vi "Logic for Default Case.vi"(11 "error in (no error)":errorcluster) -> (15 "error out":errorcluster)   [LabVIEW 2021, in "Migrator.lvlib"]
uses:
  Migrator.lvlib
  <vilib>/Utility/traverseref.llb/TRef TravTarget.ctl
  <vilib>/Utility/traverseref.llb/VI Scripting - Traverse.lvlib
  Path Functions/Path Functions.lvlib
  Migrator Reusables/Migrator Reusables.lvlib
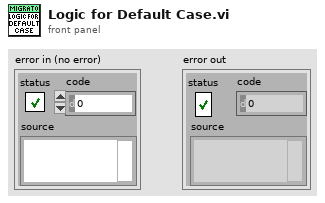
[diagram p1: front panel]
types:
  T1 = typedef "TRef TravTarget.ctl" = enum16{"FP", "BD", "Other"}
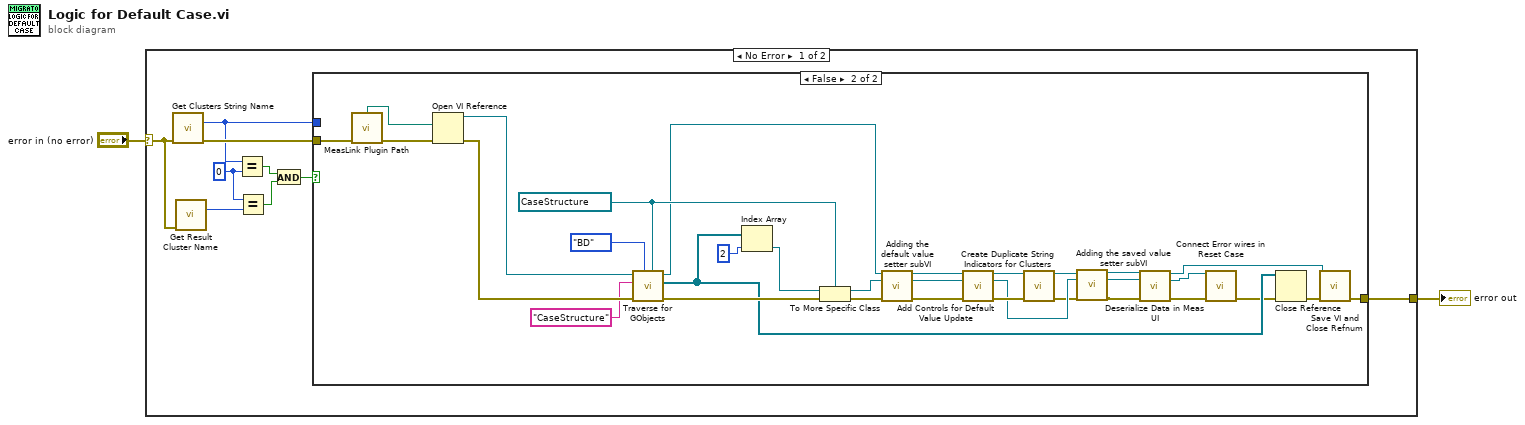
[diagram p0: block diagram]
diagram:
  n1 = case shown="No Error" "error in (no error)" {
    selector: "error in (no error)" -> [w10 w45]
    tunnel: [w11 w45] -> w2
    frame No Error {
      w7 = 0 ("y")
      n2 = call "Get Clusters String Name.vi"("error in (no error)"=w10) -> ("Array Size"=w8:i32, "error out"=w9:errorcluster)  [unwired: 12 in, 1 out]
      n3 = call "Get Result Cluster Name.vi"("error in (no error)"=w10) -> ("Array Size"=w6:i32)  [unwired: 12 in, 2 out]
      n4 = Equal?(x=w8, y=w7) -> (x = y?=w5:bool)
      n5 = Equal?(x=w7, y=w6) -> (x = y?=w4:bool)
      n6 = And(x=w5, y=w4) -> (x .and. y?=w3:bool)
      n7 = case shown="False" w3 {
        tunnel: [w12 w37] -> w11
        tunnel: w9 -> [w12 w13]
        tunnel: w8 -> [_ _]
        frame True {
        }
        frame False {
          w40 = refnum<vi> refnum ("Other Refnum")
          n8 = call "MeasLink Plugin Path.vi"("error in (no error)"=w13) -> ("Measurement UI"=w34:path, "error out"=w44:errorcluster)  [unwired: 2 in, 11 out]
          n9 = Open VI Reference(vi path=w34, error in (no error)=w44) -> (vi reference=w31:refnum<vi>, error out=w43:errorcluster)  [unwired: 4 in]
          n10 = call <vilib>:"Traverse for GObjects.vi"("Other Refnum"=w40, "Traverse Target"=TRef_TravTarget."BD", "error in (no error)"=w43, "Class Name"="CaseStructure", "VI Refnum"=w31) -> ("error out"=w39:errorcluster, "References"=w23:refnum<vi>[], "dup VI Refnum"=w21:refnum<vi>)  [unwired: 3 in, 1 out]
          n11 = Index Array(array=w23, index=2) -> (element=w35:refnum<vi>)
          n12 = To More Specific Class(target class=w40, reference=w35, error in=w39) -> (specific class reference=w33:refnum<vi>, error out=w38:errorcluster)
          n13 = call "Adding the default value setter subVI.vi"("VI in"=w21, "Case Sel Refnum"=w33, "error in (no error)"=w38) -> ("VI Out"=w30:refnum<vi>, "Case Sel Refnum Out"=w17:refnum<vi>, "error out"=w18:errorcluster)  [unwired: 10 in]
          n14 = call "Add Controls for Default Value Update.vi"("VI Refnum"=w30, "Case Sel Refnum"=w17, "error in (no error)"=w18) -> ("VI Refnum Out"=w29:refnum<vi>, "Case Sel Refnum Out"=w27:refnum<vi>, "error out"=w32:errorcluster)  [unwired: 10 in]
          n15 = call "Create Duplicate String Indicators for Clusters.vi"("UI VI Ref"=w29, "error in (no error)"=w32) -> ("UI VI Ref Out"=w28:refnum<vi>, "error out"=w19:errorcluster)  [unwired: 12 in]
          n16 = call "Adding the saved value setter subVI.vi"("VI in"=w28, "Case Sel Refnum"=w27, "error in (no error)"=w19) -> ("VI Out"=w26:refnum<vi>, "Case Sel Refnum Out"=w25:refnum<vi>, "error out"=w20:errorcluster)  [unwired: 10 in]
          n17 = call "Deserialize Data in Meas UI.vi"("VI Refnum"=w26, "Case Sel Refnum"=w25, "error in (no error)"=w20) -> ("VI Refnum Out"=w24:refnum<vi>, "Case Sel Refnum Out"=w16:refnum<vi>, "error out"=w14:errorcluster)  [unwired: 10 in]
          n18 = call "Connect Error wires in Reset Case.vi"("Case Sel Refnum"=w16, "error in (no error)"=w14) -> ("error out"=w15:errorcluster)  [unwired: 12 in, 1 out]
          n19 = Close Reference(reference=w23, error in (no error)=w15) -> (error out=w22:errorcluster)
          n20 = call "Save VI and Close Refnum.vi"("VI Refnum"=w24, "error in"=w22) -> ("error out"=w37:errorcluster)  [unwired: 13 in]
        }
      }
    }
    frame Error {
    }
  }
  "error out" <- w2
